vi "mod_Phase Noise Fit.vi"(0 "single sided phase noise density":cluster{"f0":dbl, "df":dbl, "magnitude":dbl[]} {"f0" format="%.2p"; "df" format="%.2p"; "magnitude" format="%.2p"}, 11 "error in (no error)":errorcluster) -> (4 "raw phase noise":cluster{"f0":dbl, "df":dbl, "magnitude":dbl[]} {"f0" format="%.2p"; "df" format="%.2p"; "magnitude" format="%.2p"}, 6 "fitted phase noise":cluster{dbl, dbl, dbl[]} {"?" format="%.2f"; "?" format="%.2f"; "?" format="%.2f"}, 15 "error out":errorcluster)   [LabVIEW 2020, in "niAMT.lvlib"]
uses:
  <vilib>/addons/Modulation/niAMT.lvlib
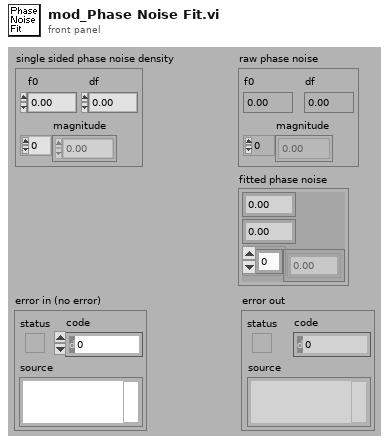
[diagram p1: front panel]
types:
  T1 = cluster{"Ramp Pattern":dbl[], "phase noise":dbl[]}[]
  T2 = cluster{"Ramp Pattern":dbl[], "phase noise":dbl[]}
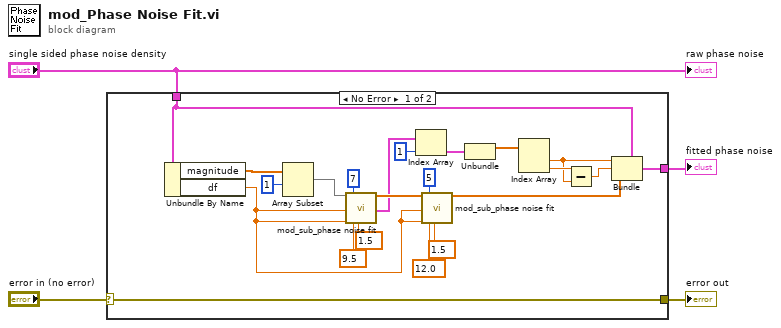
[diagram p0: block diagram]
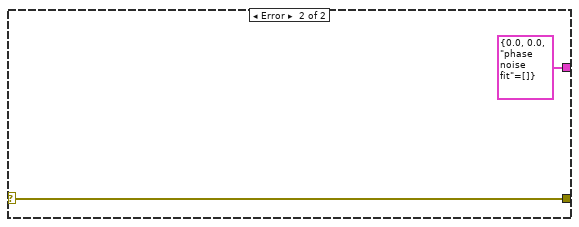
[diagram p2: hidden frame]
diagram:
  n1 = case shown="No Error" "error in (no error)" {
    selector: "error in (no error)" -> [w6 w28]
    tunnel: [w14 cluster{dbl, dbl, "phase noise fit":dbl[]} {0.0, 0.0, "phase noise fit"=[]}] -> w4
    tunnel: "single sided phase noise density" -> [w5 _]
    tunnel: [w6 w28] -> w1
    frame No Error {
      n2 = Unbundle By Name(w5) -> ("magnitude"=w8:dbl[], "df"=w10:dbl)
      n3 = Array Subset(array=w8, index=1) -> (w7:dbl[])  [unwired: 1 in]
      n4 = call <vilib>:"mod_sub_phase noise fit.vi"("raw phase noise in"=w7, "f0"=w10, "df"=w10, "polynomial order"=7, "Section at what multiples?"=9.5, "multiple buffer?"=1.5) -> ("phase noise fit"=w22:dbl[], "phase noise plots"=w20:T1)  [unwired: 1 in, 11 out]
      n5 = Index Array(array=w20, index=1) -> (element=w17:T2)
      n6 = call <vilib>:"mod_sub_phase noise fit.vi"("raw phase noise in"=w22, "f0"=w10, "df"=w10, "polynomial order"=5, "Section at what multiples?"=12.0, "multiple buffer?"=1.5) -> ("phase noise fit"=w13:dbl[])  [unwired: 1 in, 12 out]
      n7 = Unbundle(w17) -> ("Ramp Pattern"=w16:dbl[])  [unwired: 1 out]
      n8 = Index Array(array=w16) -> (element #1=w11:dbl, element #2=w15:dbl)  [unwired: 2 in]
      n9 = Subtract(x=w15, y=w11) -> (x-y=w12:dbl)
      n10 = Bundle(cluster=w5, "f0"=w11, "df"=w12, "magnitude"=w13) -> (w14:cluster{"f0":dbl, "df":dbl, "magnitude":dbl[]})
    }
    frame Error {
    }
  }
  "fitted phase noise" <- w4
  "error out" <- w1
  "raw phase noise" <- "single sided phase noise density"
